vi "AI Comtinuous Engine Testing.vi"(8 "error in (no error)":errorcluster) -> (0 "error out":errorcluster)   [LabVIEW 2013]
doc: "Copyright © 2005, Soliton Technologies.\nAll rights reserved."
uses:
  Controls/SLL DE Circular Buffer Options.ctl
  Controls/SLL DE Circular Buffer Pointers List.ctl
panel:
  out "x != y?":bool
  out "Waveform Chart":sgl[][](graph)
  out "Time":i32
  out "Data":i32
  in  "stop":bool
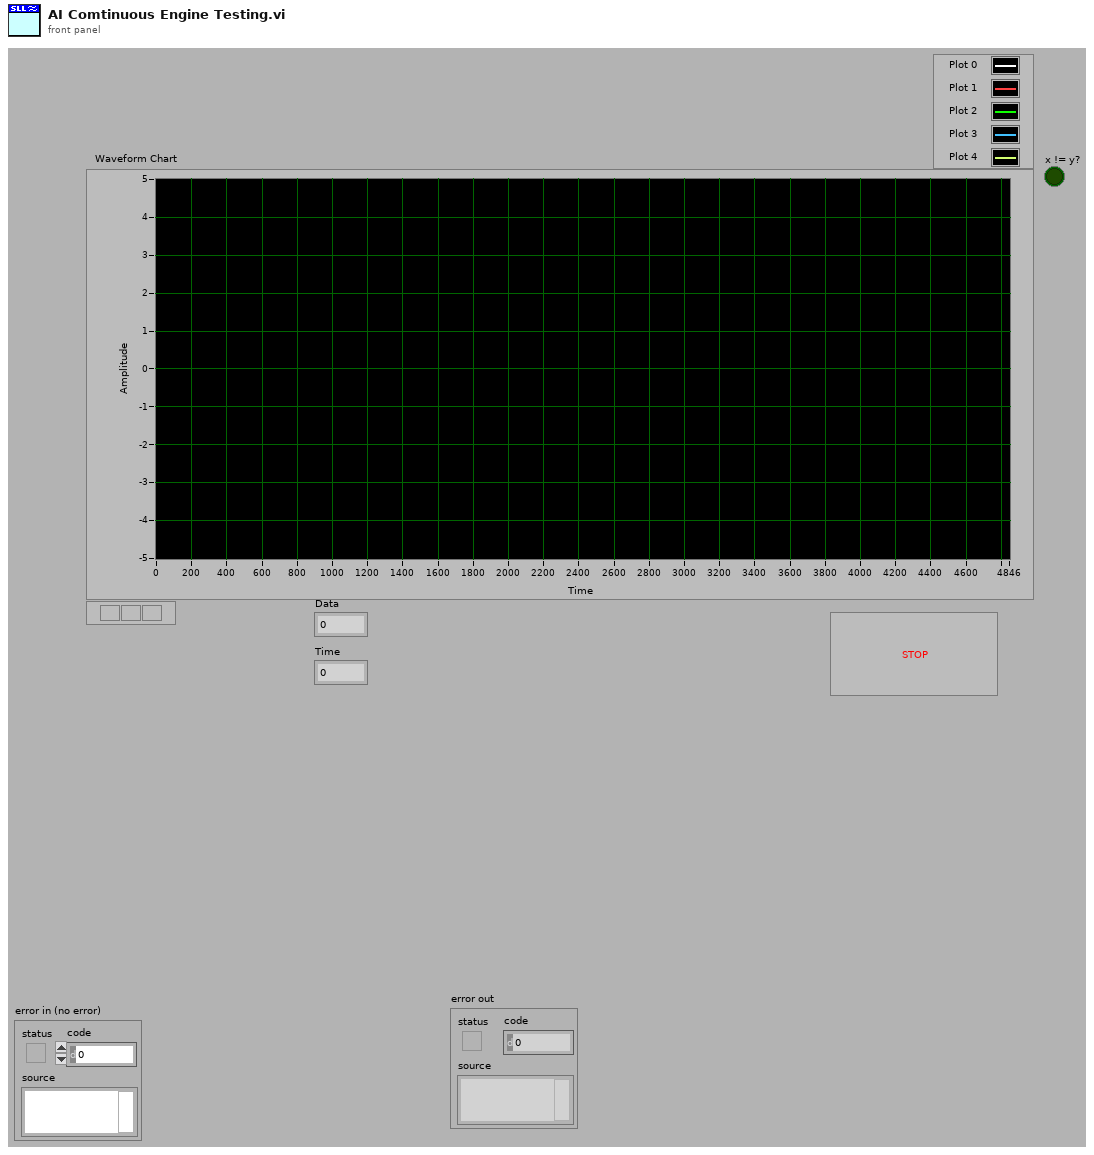
[diagram p1: front panel]
types:
  T1 = typedef "SLL DE Circular Buffer Pointers List.ctl" = enum16{"Graph Pointer", "File Log Pointer", "Pointer 3", "Pointer 4"}
  T2 = typedef "SLL DE Circular Buffer Options.ctl" = enum16{"Initialize", "Init Pointer X", "Write", "Read Single Value", "Read Pointer X (Multi Value)", "Clear Data"}
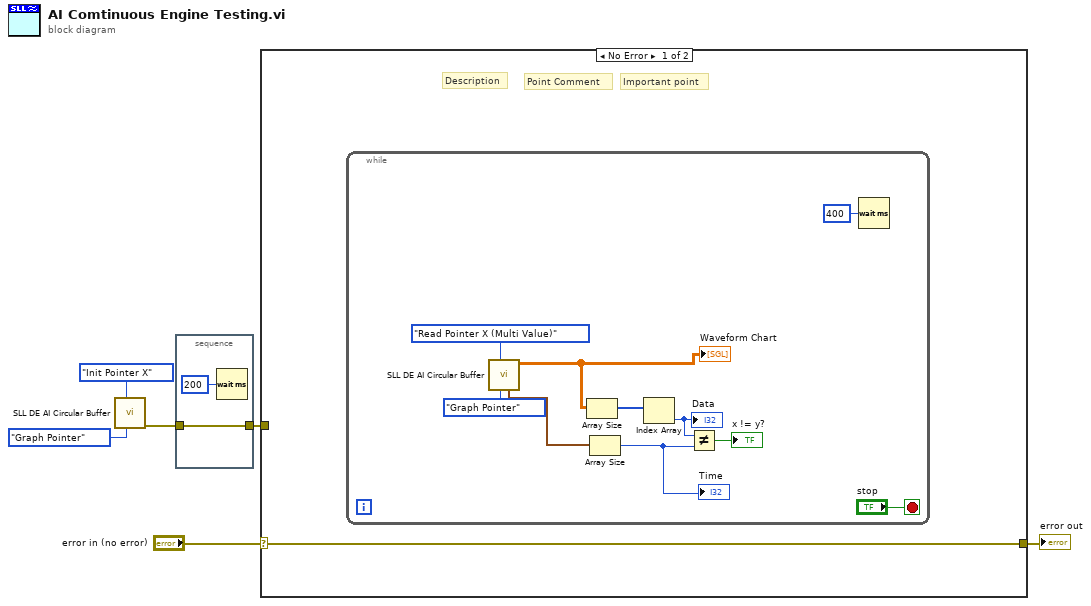
[diagram p0: block diagram]
diagram:
  n1 = call "SLL DE AI Circular Buffer.vi"("Pointers"=SLL_DE_Circular_Buffer_Pointers_List."Graph Pointer", "Options"=SLL_DE_Circular_Buffer_Options."Init Pointer X" ("AI Option")) -> ("error Out"=w2:errorcluster)  [unwired: 4 in, 5 out]
  n2 = stacked-sequence {
    tunnel: w2 -> [w8]
    tunnel: [w8] -> w1
    frame #0 {
      n3 = Wait (ms)(milliseconds to wait=u32 200) -> ()  [unwired: 1 out]
    }
  }
  n4 = case shown="No Error" "error in (no error)" {
    selector: "error in (no error)" -> [w9 w20]
    tunnel: [w9 w20] -> w5
    tunnel: w1 -> [_ _]
    frame No Error {
      # "Point Comment"
      # "Important point"
      # "Description"
      n5 = while {
        stop <- "stop" stop-if-true
        n6 = call "SLL DE AI Circular Buffer.vi"("Pointers"=SLL_DE_Circular_Buffer_Pointers_List."Graph Pointer", "Options"=SLL_DE_Circular_Buffer_Options."Read Pointer X (Multi Value)" ("AI Option")) -> ("Output Data"=w15:sgl[][], "Multi Time Stamp"=w10:timestamp[])  [unwired: 4 in, 4 out]
        "Waveform Chart" <- w15
        n7 = Array Size(array=w15) -> (size(s)=w16:i32[])
        n8 = Array Size(array=w10) -> (size(s)=w12:i32)
        "Time" <- w12
        n9 = Index Array(array=w16) -> (element=w13:i32)  [unwired: 1 in]
        "Data" <- w13
        n10 = Not Equal?(x=w13, y=w12) -> (x != y?=→"x != y?":bool)
        n11 = Wait (ms)(milliseconds to wait=u32 400) -> ()  [unwired: 1 out]
      }
    }
    frame Error {
    }
  }
  "error out" <- w5
